vi "Save TDMS.vi"(8 "error in (no error)":errorcluster, 9 "GlobalData":T2, 10 "Data":variant, 11 "tdms file in":refnum<k34>) -> (0 "error out":errorcluster, 3 "tdms file out":refnum<k34>)   [LabVIEW 2024]
doc: "This vi used to log measurements into tdms file"
uses:
  controls/GlobalData.ctl
  controls/Units.ctl
  <userlib>/_OpenG.lib/lvdata/lvdata.llb/openg_variant.lvlib
panel:
  in  "Units Settings":T1={"Pressure"=enum."Pa", "Temperature"=enum."F", "Salinity"=enum."ppt", "Weight"=enum."ib"}
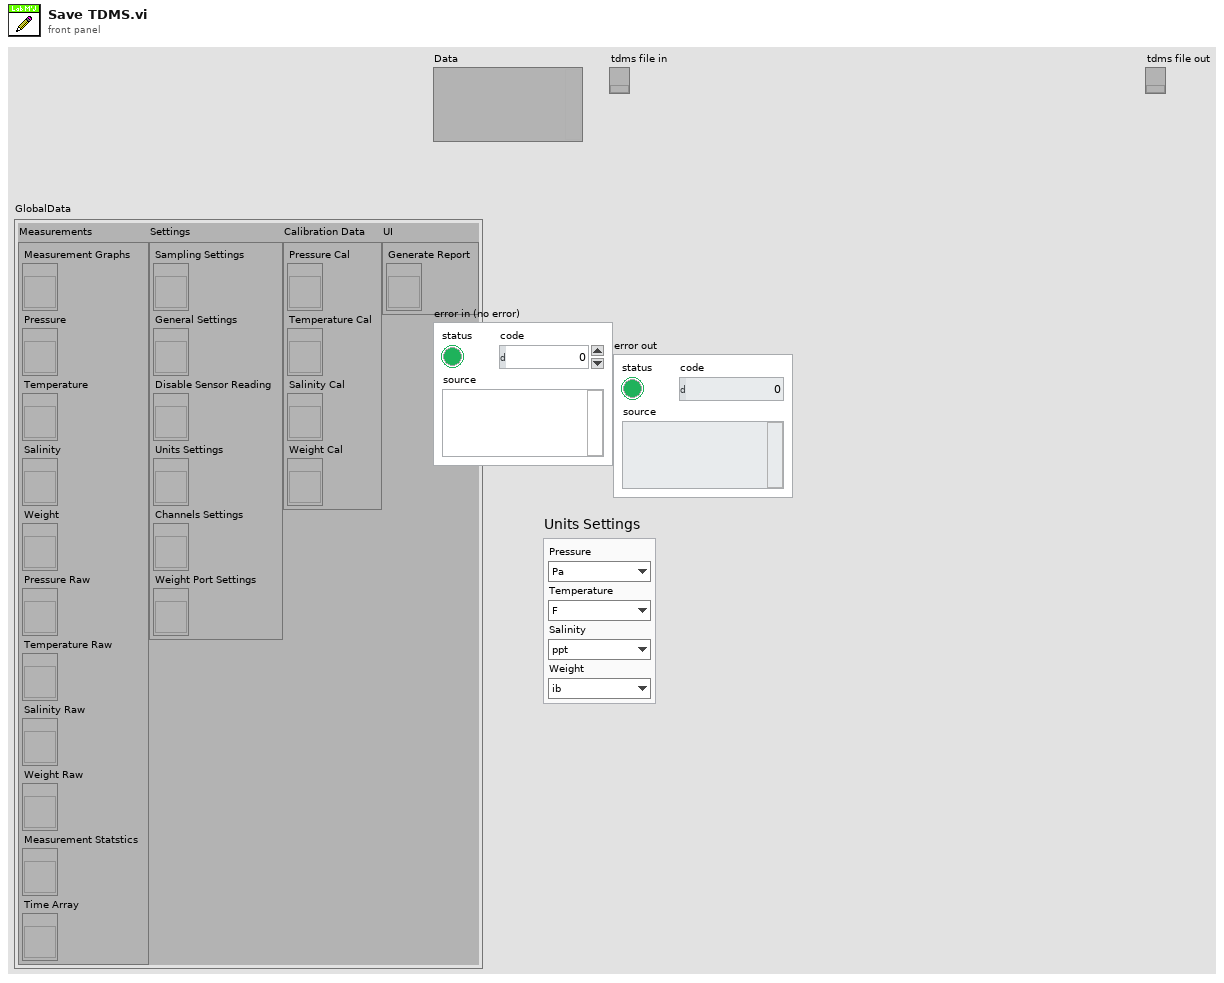
[diagram p1: front panel]
types:
  T1 = typedef "Units.ctl" = cluster{"Pressure":enum16{"PSI", "Bar", "atm", "Pa"}, "Temperature":enum16{"C", "K", "F"}, "Salinity":enum16{"ppm", "ppt", "PSU"}, "Weight":enum16{"Kg", "g", "oz", "ib"}}
  T2 = typedef "GlobalData.ctl" = cluster{"Measurements":cluster{"Measurement Graphs":refnum<vi>, "Pressure":refnum<vi>, "Temperature":refnum<vi>, "Salinity":refnum<vi>, "Weight":refnum<vi>, "Pressure Raw":refnum<vi>, "Temperature Raw":refnum<vi>, "Salinity Raw":refnum<vi>, "Weight Raw":refnum<vi>, "Measurement Statstics":refnum<vi>, "Time Array":refnum<vi>}, "Settings":cluster{"Sampling Settings":refnum<vi>, "General Settings":refnum<vi>, "Disable Sensor Reading":refnum<vi>, "Units Settings":refnum<vi>, "Channels Settings":refnum<vi>, "Weight Port Settings":refnum<vi>}, "Calibration Data":cluster{"Pressure Cal":refnum<vi>, "Temperature Cal":refnum<vi>, "Salinity Cal":refnum<vi>, "Weight Cal":refnum<vi>}, "UI":cluster{"Generate Report":refnum<vi>}}
  T3 = cluster{"Reading Time (ms)":u64, "Graph Time ":u16}
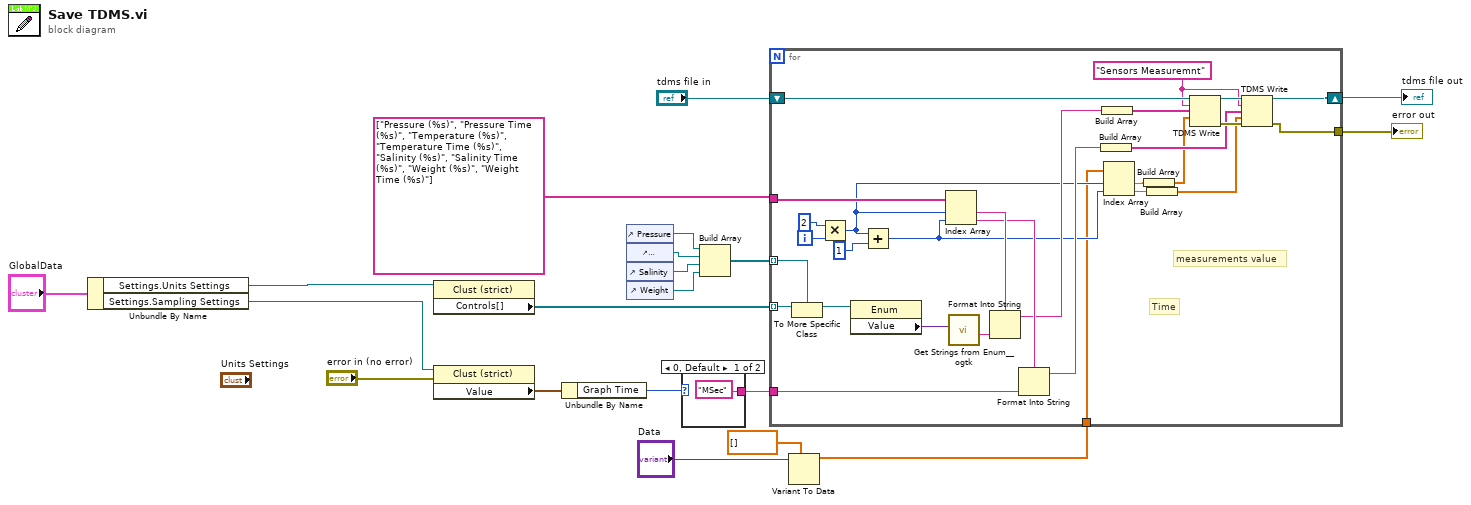
[diagram p0: block diagram]
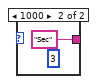
[diagram p2: hidden frame]
diagram:
  n1 = Unbundle By Name("GlobalData") -> ("Settings.Units Settings"=w19:refnum<vi>, "Settings.Sampling Settings"=w16:refnum<vi>)
  n2 = property on="Property Node" class="Clust (strict)"(reference=w19) -> ("Controls[]"=w18:refnum<vi>[])  [unwired: 1 in, 2 out]
  n3 = property on="Property Node" class="Clust (strict)"(reference=w16, error in="error in (no error)") -> ("Value"=w17:T3)  [unwired: 2 out]
  n4 = Unbundle By Name(w17) -> ("Graph Time"=w14:u16)
  n5 = control-ref of="Pressure"() -> (w6:refnum<vi>)
  n6 = control-ref of="Temperature"() -> (w7:refnum<vi>)
  n7 = control-ref of="Salinity"() -> (w8:refnum<vi>)
  n8 = control-ref of="Weight"() -> (w9:refnum<vi>)
  n9 = case shown="0, Default" w14 {
    tunnel: ["MSec" ("X Scale.Name Label.Text") "Sec" ("X Scale.Name Label.Text")] -> w15
    frame 0, Default {
    }
    frame 1000 {
      (unwired) u64 3 ("Reading Time (ms)")
    }
  }
  n10 = Build Array(w6, w7, w8, w9) -> (w5:refnum<vi>[])
  n11 = Variant To Data(type=dbl[] [] ("appended array"), Variant="Data") -> (data=w4:dbl[])  [unwired: 1 in, 1 out]
  n12 = for {
    tunnel: w18 -> [w51] mode=indexing
    tunnel: w15 -> [w47]
    tunnel: string[] ["Pressure (%s)", "Pressure Time (%s)", "Temperature (%s)", "Temperature Time (%s)", "Salinity (%s)", "Salinity Time (%s)", "Weight (%s)", "Weight Time (%s)"] ("channel name(s) in (Untitled)") -> [w46]
    tunnel: w5 -> [w41] mode=indexing
    shift-right: [w36] -> w2
    shift-left: "tdms file in" -> [w40]
    tunnel: w4 -> [w23]
    tunnel: [w24] -> w1
    i -> [w25]
    w37 = "Sensors Measuremnt" ("group name")
    # "Time"
    # "measurements value"
    n13 = To More Specific Class(target class=w41, reference=w51) -> (specific class reference=w50:refnum<vi>)  [unwired: 1 in, 1 out]
    n14 = Multiply(x=2, y=w25) -> (x*y=w31:i32)
    n15 = property on="Property Node" class="Enum"(reference=w50) -> ("Value"=w49:variant)  [unwired: 1 in, 2 out]
    n16 = Add(x=w31, y=1) -> (x+y=w30:i32)
    n17 = Index Array(array=w46, index #1=w31, index #2=w30) -> (element #1=w44:string, element #2=w42:string)
    n18 = call <userlib>:"Get Strings from Enum__ogtk.vi"("Enum"=w49) -> ("String Value"=w48:string)  [unwired: 7 in, 3 out]
    n19 = Format Into String(format string=w44, w48) -> (resulting string=w35:string)  [unwired: 2 in, 1 out]
    n20 = Format Into String(format string=w42, w47) -> (resulting string=w33:string)  [unwired: 2 in, 1 out]
    n21 = Build Array(w33) -> (w32:string[])
    n22 = Build Array(w35) -> (w34:string[])
    n23 = Index Array(array=w23, index #1=w31, index #2=w30) -> (element #1=w29:dbl, element #2=w27:dbl)
    n24 = Build Array(w29) -> (w28:dbl[])
    n25 = Build Array(w27) -> (w26:dbl[])
    n26 = TDMS Write(0:w40, 5:w37, 7:w34, 9:w28) -> (4:w39:refnum<k34>, 15:w38:errorcluster)  [unwired: 2 in, 2 out]
    n27 = TDMS Write(0:w39, 5:w37, 7:w32, 9:w26, 11:w38) -> (4:w36:refnum<k34>, 15:w24:errorcluster)  [unwired: 1 in, 2 out]
  }
  "tdms file out" <- w2
  "error out" <- w1
